vi "Endpoint Connected.vi"(8 "error in":errorcluster, 10 "Endpoint":refnum<class "Message Enqueuer.lvclass">, 11 "CRIO MSS Test Actor in":refnum<class "CRIO MSS Test Actor.lvclass">) -> (0 "error out":errorcluster, 3 "CRIO MSS Test Actor out":refnum<class "CRIO MSS Test Actor.lvclass">)   [LabVIEW 2023, in "CRIO MSS Test Actor.lvlib" / "CRIO MSS Test Actor.lvclass"]
doc: "Override this method to specify how the receiving actor responds to a Connected message from a nested endpoint actor."
uses:
  CRIO MSS Test Actor.lvclass
  <vilib>/ActorFramework/Message Enqueuer/Message Enqueuer.lvclass
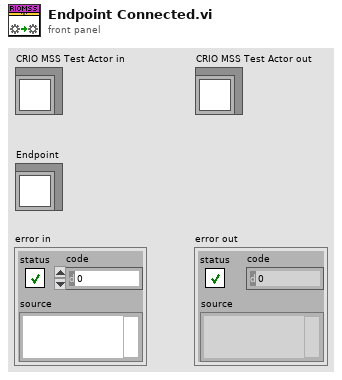
[diagram p1: front panel]
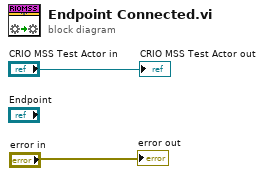
[diagram p0: block diagram]
diagram:
  "error out" <- "error in"
  "CRIO MSS Test Actor out" <- "CRIO MSS Test Actor in"
